vi "Copy Memory Address to Image (ARGB).vi"(8 "error in (no error)":errorcluster, 10 "ARGB Image Destination":T1, 11 "Source":T2) -> (0 "error out":errorcluster, 3 "ARGB Image Destination (Duplicate)":T1)   [LabVIEW 2020, in "image.lvlib"]
uses:
  image.lvlib
  Raw Memory Information.ctl
  Raw Memory Information Dimension.ctl
  ARGB Image.ctl
  e0109ec8-11ee-4a07-aeee-d632e4e22c38.vi
  common/Module Path.vi
  <vilib>/Utility/error.llb/Error Cluster From Error Code.vi
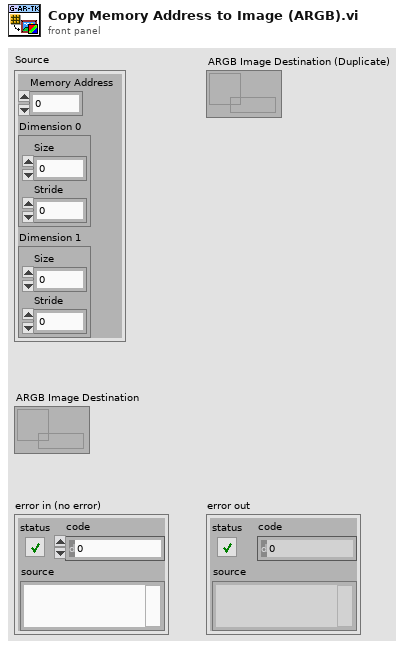
[diagram p1: front panel]
types:
  T1 = typedef "image.lvlib/ARGB Image.ctl" = refnum<data-value>
  T2 = typedef "image.lvlib/Raw Memory Information.ctl" = cluster{"Memory Address":u64, "Dimension 0":T3, "Dimension 1":T3}
  T3 = typedef "image.lvlib/Raw Memory Information Dimension.ctl" = cluster{"Size":u16, "Stride":u32}
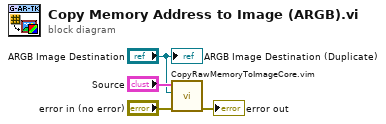
[diagram p0: block diagram]
diagram:
  n1 = call "CopyRawMemoryToImageCore.vim"("error in (no error)"="error in (no error)", "Dst"="ARGB Image Destination", "Source"="Source") -> ("error out"=→"error out":errorcluster)  [unwired: 8 in]
  "ARGB Image Destination (Duplicate)" <- "ARGB Image Destination"
